vi "LED Init.vi"(8 "error in (no error)":errorcluster) -> (0 "error out":errorcluster, 3 "LEDs":T1)   [LabVIEW 2020]
uses:
  <vilib>/High Genius/HG_WSI_Tookit/Dependencies/Library/Digital Input and Output/Digital Input and Output.lvclass
  C:/Program Files (x86)/National Instruments/LabVIEW 2020/vi.lib/High Genius/HG_WSI_Tookit/Dependencies/Library/HG_LIB/HG_LIB.lvclass
  <vilib>/High Genius/HG_WSI_Tookit/Dependencies/Library/HG_LIB/HG_LIB.lvclass
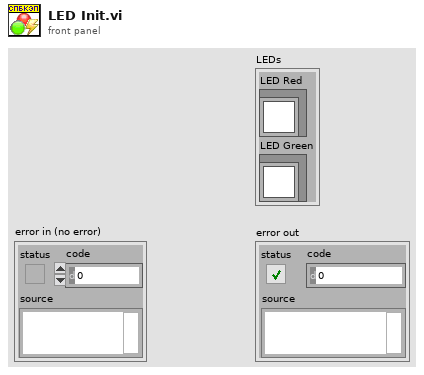
[diagram p1: front panel]
types:
  T1 = cluster{"LED Red":refnum<class "Digital Input and Output.lvclass">, "LED Green":refnum<class "Digital Input and Output.lvclass">}
  T2 = enum16{"0", "1", "2", "3", "4", "5", "6", "7", "8", "9", "10", "11", "12", "13", "14", "15", "16", "17", "18", "19", "20", "21", "22", "23", "24", "25"}
  T3 = enum16{"DI", "DO", "AI", "Pulse", "PWM", "ISQ", "ENC", "CAN", "IIC", "IMU"}
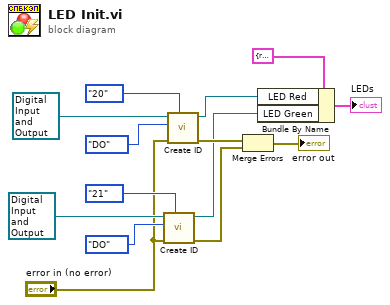
[diagram p0: block diagram]
diagram:
  n1 = call <vilib>:"Create ID.vi"("NO"=T2."21", "error in (no error)"="error in (no error)", "Function"=T3."DO", "HG_LIB in"=refnum<class "Digital Input and Output.lvclass"> refnum ("VMX Library.lvlib:Digital Input and Output.lvclass")) -> ("error out"=w7:errorcluster, "HG_LIB out"=w4:refnum<class "Digital Input and Output.lvclass">)  [unwired: 6 in]
  n2 = call <vilib>:"Create ID.vi"("NO"=T2."20", "error in (no error)"="error in (no error)", "Function"=T3."DO", "HG_LIB in"=refnum<class "Digital Input and Output.lvclass"> refnum ("VMX Library.lvlib:Digital Input and Output.lvclass")) -> ("error out"=w8:errorcluster, "HG_LIB out"=w3:refnum<class "Digital Input and Output.lvclass">)  [unwired: 6 in]
  n3 = Merge Errors(w8, w7) -> (→"error out":errorcluster)
  n4 = Bundle By Name(cluster=T1 {"LED Red"=refnum, "LED Green"=refnum} ("HG_LIB out"), "LED Red"=w3, "LED Green"=w4) -> (→"LEDs":T1)
